vi "Dead Band.vi"(2 "Axis 2 In":dbl, 3 "Axis 1 In":dbl, 4 "Dead Band":dbl=0.25) -> (0 "Axis 2 Out":dbl, 1 "Axis 1 Out":dbl)   [LabVIEW 2012]
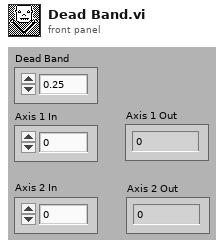
[diagram p1: front panel]
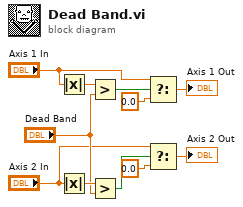
[diagram p0: block diagram]
diagram:
  n1 = Absolute Value(x="Axis 1 In") -> (abs(x)=w8:dbl)
  n2 = Absolute Value(x="Axis 2 In") -> (abs(x)=w5:dbl)
  n3 = Greater?(x=w8, y="Dead Band") -> (0:w7:bool)
  n4 = Greater?(x=w5, y="Dead Band") -> (0:w6:bool)
  n5 = Select(t="Axis 1 In", s=w7, f=0.0) -> (s? t:f=→"Axis 1 Out":dbl)
  n6 = Select(t="Axis 2 In", s=w6, f=0.0) -> (s? t:f=→"Axis 2 Out":dbl)
